vi "HEWH Sample Received Date.vi"(8 "error in (no error)":errorcluster, 11 "date time rec":T1) -> (0 "error out":errorcluster, 3 "Sample received Date":string)   [LabVIEW 2019]
uses:
  <vilib>/Utility/miscctls.llb/LVDateTimeRec.ctl
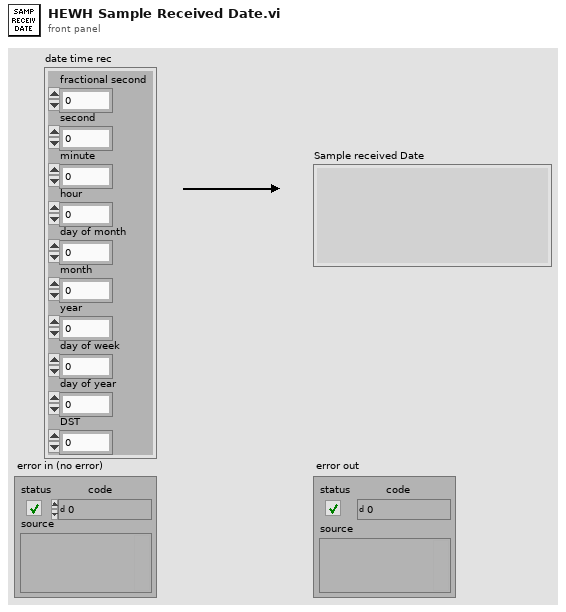
[diagram p1: front panel]
types:
  T1 = typedef "LVDateTimeRec.ctl" = cluster{"fractional second":dbl, "second":i32, "minute":i32, "hour":i32, "day of month":i32, "month":i32, "year":i32, "day of week":i32, "day of year":i32, "DST":i32}
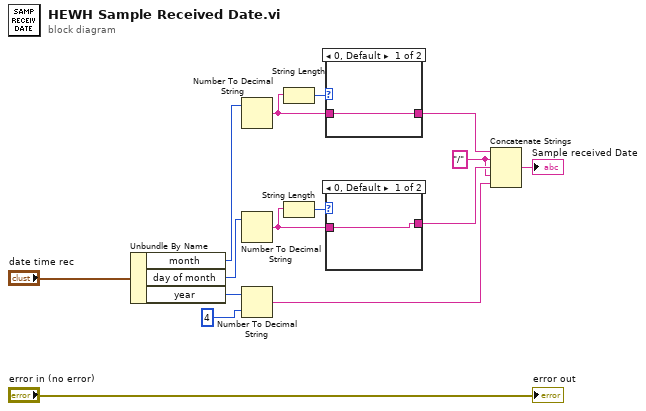
[diagram p0: block diagram]
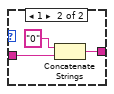
[diagram p2: hidden frame]
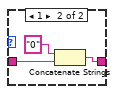
[diagram p3: hidden frame]
diagram:
  w7 = "/" ("string")
  n1 = Unbundle By Name("date time rec") -> ("month"=w3:i32, "day of month"=w4:i32, "year"=w5:i32)
  n2 = Number To Decimal String(number=w3) -> (decimal integer string=w11:string)  [unwired: 1 in]
  n3 = Number To Decimal String(number=w4) -> (decimal integer string=w13:string)  [unwired: 1 in]
  n4 = Number To Decimal String(number=w5, width (-)=i16 4) -> (decimal integer string=w8:string)
  n5 = String Length(string=w11) -> (length=w10:i32)
  n6 = String Length(string=w13) -> (length=w12:i32)
  n7 = case shown="0, Default" w10 {
    tunnel: w11 -> [w16 w18]
    tunnel: [w16 w17] -> w15
    frame 0, Default {
    }
    frame 1 {
      n8 = Concatenate Strings("0" ("string"), w18) -> (w17:string)
    }
  }
  n9 = case shown="0, Default" w12 {
    tunnel: w13 -> [w20 w22]
    tunnel: [w20 w21] -> w14
    frame 0, Default {
    }
    frame 1 {
      n10 = Concatenate Strings("0" ("string"), w22) -> (w21:string)
    }
  }
  n11 = Concatenate Strings(w15, w7, w14, w7, w8) -> (→"Sample received Date":string)
  "error out" <- "error in (no error)"
